vi "Invalid Architecture--error.vi"() -> (0 "error out":errorcluster)   [LabVIEW 2025]
doc: "Indicates that the specified architecture is invalid. It must be 64 or 32."
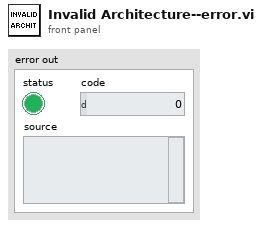
[diagram p1: front panel]
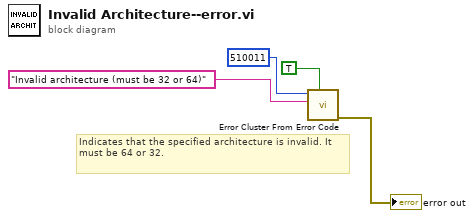
[diagram p0: block diagram]
diagram:
  # "Indicates that the specified architecture is invalid. It must be 64 or 32."
  n1 = call <vilib>:"Error Cluster From Error Code.vi"("show call chain? (False)"=TRUE, "error message (\"\")"="Invalid architecture (must be 32 or 64)" ("error message (\"\")"), "error code (0)"=510011) -> ("error out"=→"error out":errorcluster)  [unwired: 6 in]
